vi "PID_TUNING.vi"() -> ()   [LabVIEW 2014]
doc: "This example performs writes and reads on a serial port, as directed by the user. You can press the Write and Read buttons, and change the Read Count, while the example is running.\n\nThe parameters set for the serial port must match the parameters of the connected instrument or device. In this example, the Read Count parameter specifies the number of bytes that the serial port reads. If there were more bytes at the port than the specified number, those bytes would not be read. If there were less bytes at the port than the specified number, you would receive a timeout error.\n\nThis example expands upon the flow control options for XON and XOFF, allowing the user to choose those control characters. Also, the user can enable or disable a termination character. Some devices require a termination character in order to identify the end of command strings. Some devices send a termination character to signify the end of data to be read. This example shows how you can end the Read operation once a termination character is detected in the buffer and/or append a termination character at the end of the Write data."
uses:
  PID Mode.ctl
  InputSimulationMode.ctl
  Serial - Settings.ctl
  Parameters.ctl
  <vilib>/Instr/_visa.llb/VISA Configure Serial Port (Instr).vi
panel:
  in  "Tab Control":enum32{"Main", "Debug"}(tab)
  out "PWM":u16(slide) scale=0.0..1023.0
  in  "Enable Commands":bool
  in  "Sync Commands":bool
  out "Input Mode Actual":T1
  in  "Input Mode":T1
  in  "COM Port":refnum<visa-resource-name>="COM1"
  in  "Stop":bool
  in  "Command Cluster":T2={"Setpoint"=0.0, "Temp C"=0.0, "Output"=0, "kP"=40.0, "kI"=1.0, "Kd"=0.1} {"Kd" scale=0.0..5.0; "kI" scale=0.0..10.0; "kP" scale=0.0..40.0; "Output" scale=0.0..961.0; "Temp C" scale=0.0..500.0; "Setpoint" scale=0.0..500.0}
  out "Setpoint":sgl(slide) scale=0.0..500.0
  out "Temp C":sgl(slide) scale=0.0..500.0
  out "Output":sgl(slide) scale=0.0..961.0
  out "kP":sgl(slide) scale=0.0..5.0
  out "kI":sgl(slide) scale=0.0..10.0
  out "Kd":sgl(slide) scale=0.0..5.0
  out "Waveform Chart":T3(graph)
  in  "PID Mode":T4
  out "PID Mode Actual":T4
  out "read buffer":string
  out "read buffer 2":string
  out "Start_of_packet":u8 format="%x"
  out "error out":errorcluster
  in  "Idle Temp C":i16
  out "Idle Temp C 2":i16
  out "Output Override":i16
  out "Simulated Tip Temp":sgl
  out "Command":string="*IDN?"
  out "adc_counts":i16
  out "Encoder Pos":i16
  out "adc_counts 2":i16
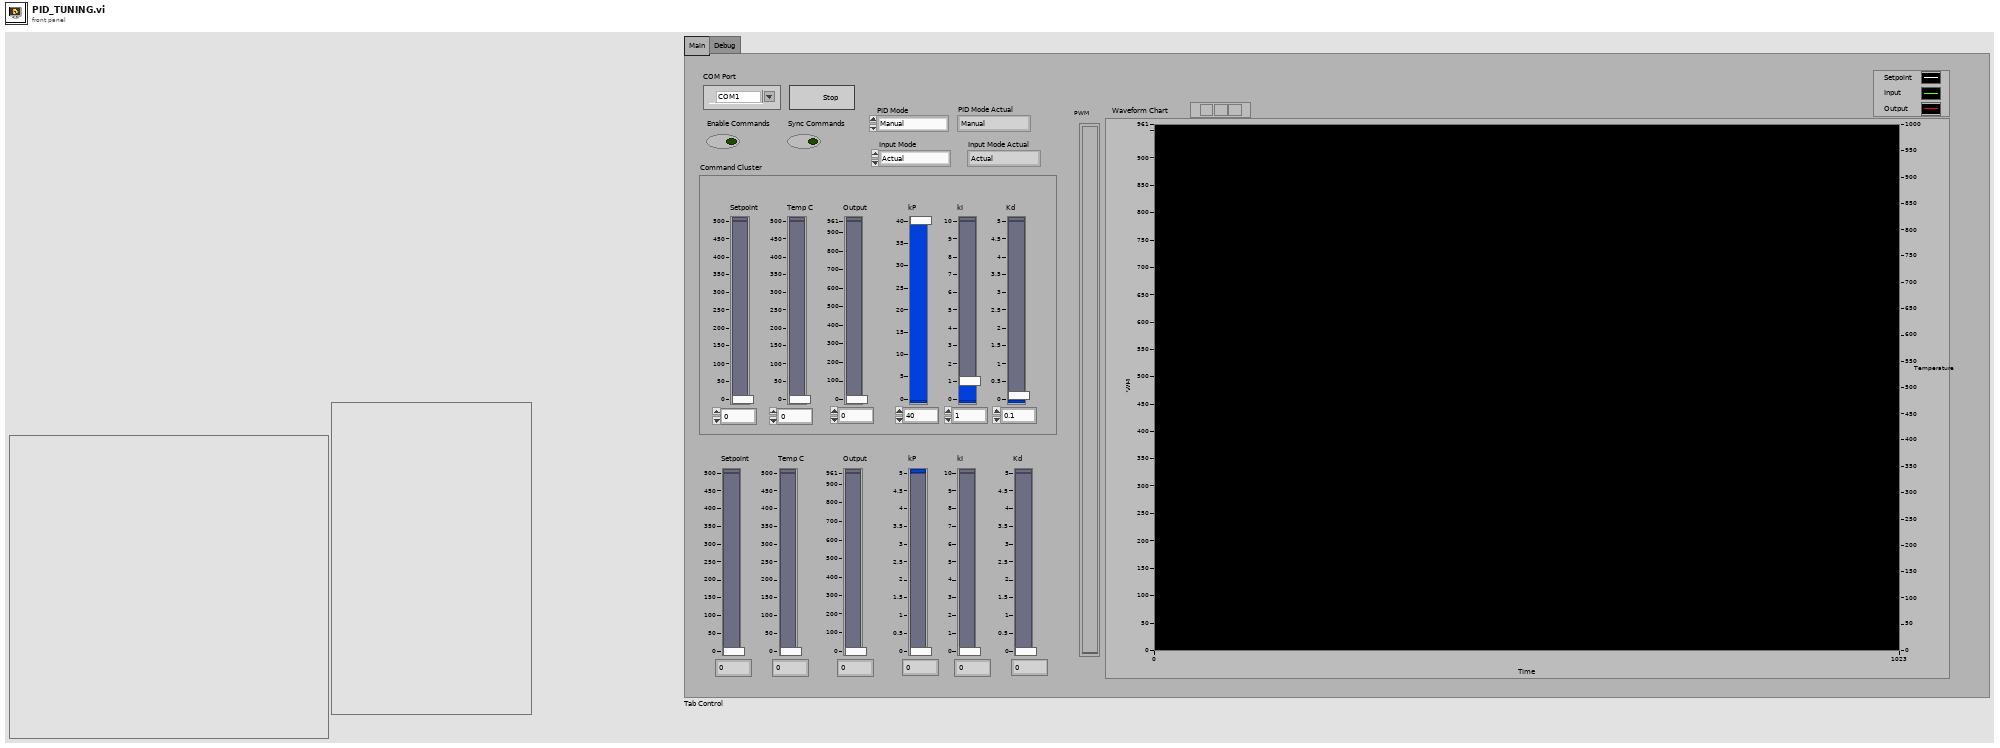
[diagram p1: front panel]
types:
  T1 = typedef "InputSimulationMode.ctl" = enum8{"Actual", "Simulated"}
  T2 = cluster{"Setpoint":sgl, "Temp C":sgl, "Output":i16, "kP":sgl, "kI":sgl, "Kd":sgl}
  T3 = cluster{"Setpoint":sgl, "Input":sgl, "Output":sgl}
  T4 = typedef "PID Mode.ctl" = enum8{"Manual", "Automatic"}
  T5 = typedef "Parameters.ctl" = cluster{"PID Mode":T4, "Input Mode":T1, "Idle Temp C":i16, "Output Override":i16, "setpoint":sgl, "kP":sgl, "kI":sgl, "kD":sgl, "Simulated Tip Temp C":sgl}
  T6 = typedef "Serial - Settings.ctl" = cluster{"baud rate":u32, "data bits":u16, "parity":enum16{"None", "Odd", "Even", "Mark", "Space"}, "stop bits":u16, "flow control":u16}
  T7 = typedef "Status.ctl" = cluster{"IO":bool[], "Encoder Pos":i16, "adapter voltage":i16, "adc_counts":i16, "adc_ic_temp_counts":i16, "current_sense_mv":i16, "PID Setpoint":sgl, "Tip Temp C":sgl, "PID Output":sgl}
  T8 = cluster{"PID Setpoint":sgl, "Tip Temp C":sgl, "PID Output":sgl}
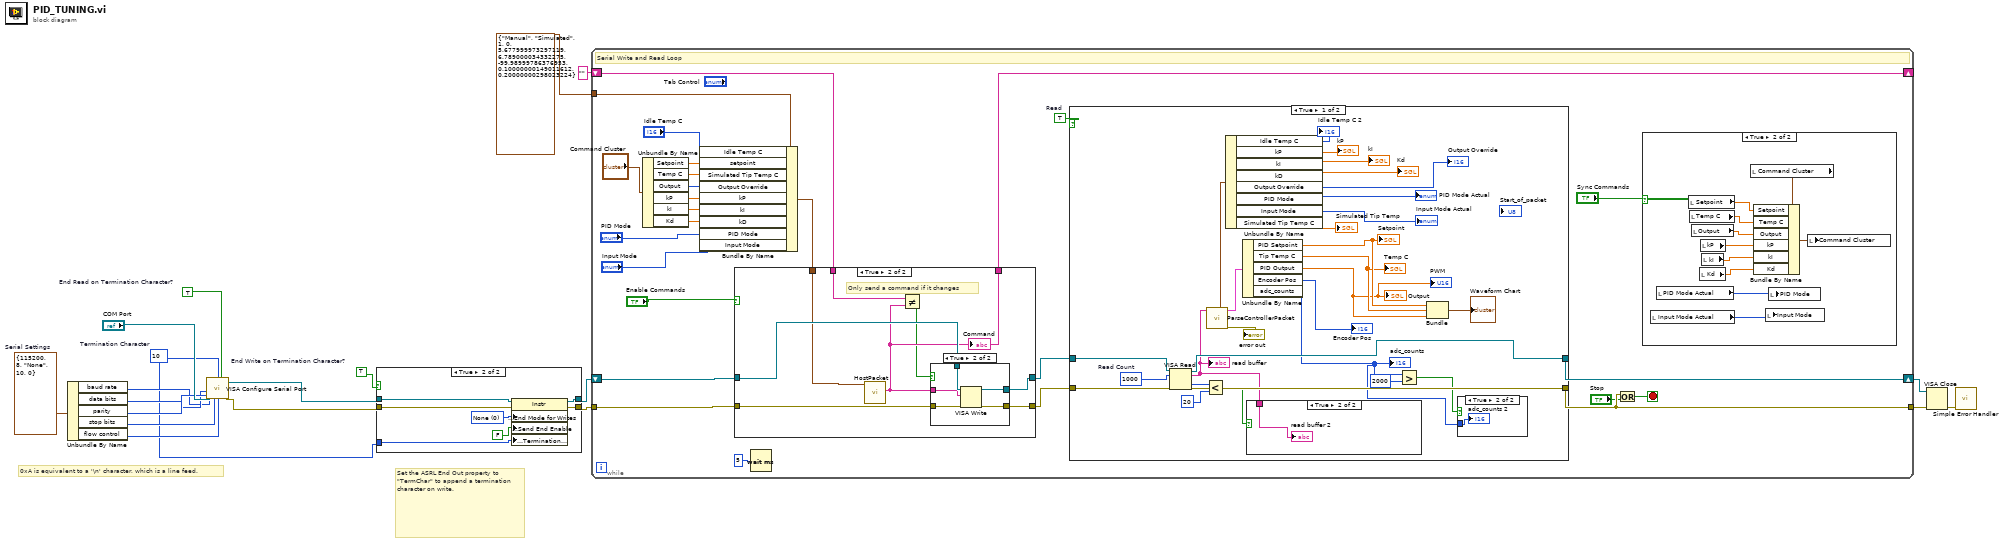
[diagram p0: block diagram]
diagram:
  w3 = u8 10  # Termination Character
  w4 = TRUE  # End Write on Termination Character?
  w11 = TRUE  # End Read on Termination Character?
  w12 = T6 {"baud rate"=115200, "data bits"=8, "parity"=enum."None", "stop bits"=10, "flow control"=0}  # Serial Settings
  # "0xA is equivalent to a '\\n' character, which is a line feed."
  # "Set the ASRL End Out property to \"TermChar\" to append a termination character on write."
  n1 = Unbundle By Name(w12) -> ("baud rate"=w13:u32, "data bits"=w14:u16, "parity"=w15:enum16{"None", "Odd", "Even", "Mark", "Space"}, "stop bits"=w16:u16, "flow control"=w7:u16)
  n2 = call-poly "VISA Configure Serial Port"("VISA resource name"="COM Port", "termination char\n(0xA = '\\n' = LF)"=w3, "Enable Termination\nChar (T)"=w11, "baud rate (9600)"=w13, "data bits (8)"=w14, "parity (0:none)"=w15, "stop bits (10: 1 bit)"=w16, "flow control (0:none)"=w7) -> ("VISA resource name out"=w17:refnum<visa-resource-name>, "error out"=w18:errorcluster)  [unwired: 2 in, 4 out]
  n3 = case shown="True" w4 {
    tunnel: w17 -> [w20 w28]
    tunnel: w18 -> [w21 w27]
    tunnel: [w20 w26] -> w5
    tunnel: [w21 w25] -> w6
    tunnel: w3 -> [_ w23]
    frame False {
    }
    frame True {
      w24 = u16 0 items=["None", "LastBit", "TermChar", "Break"] ("Serial Settings:Serial End Mode for Writes")
      n4 = property class="Instr"(reference=w28, error in=w27, "Serial Settings:End Mode for Writes"=w24, "Message Based Settings:Send End Enable"=FALSE, "Message Based Settings:Termination Character"=w23) -> (reference out=w26:refnum<visa-resource-name>, error out=w25:errorcluster)
    }
  }
  n5 = while {
    shift-right: [w54] -> w8
    shift-left: w5 -> [w53]
    tunnel: w6 -> [w52]
    tunnel: [w46] -> w9
    shift-right: [w44] -> _
    shift-left: "" ("string") -> [w43]
    tunnel: T5 {"PID Mode"=enum."Manual", "Input Mode"=enum."Simulated", "Idle Temp C"=1, "Output Override"=0, "setpoint"=5.678, "kP"=6.789, "kI"=-99.99, "kD"=0.1, "Simulated Tip Temp C"=0.2} ("Parameters") -> [w40]
    stop <- w47 stop-if-true
    w48 = TRUE  # Read
    # "Serial Write and Read Loop"
    n6 = Unbundle By Name("Command Cluster") -> ("Setpoint"=w41:sgl, "Temp C"=w39:sgl, "Output"=w38:i16, "kP"=w37:sgl, "kI"=w36:sgl, "Kd"=w35:sgl)
    n7 = Bundle By Name(cluster=w40, "Idle Temp C"="Idle Temp C", "setpoint"=w41, "Simulated Tip Temp C"=w39, "Output Override"=w38, "kP"=w37, "kI"=w36, "kD"=w35, "PID Mode"="PID Mode", "Input Mode"="Input Mode") -> (w32:T5)
    n8 = case shown="True" "Enable Commands" {
      tunnel: w53 -> [w67 w75]
      tunnel: w52 -> [w66 w74]
      tunnel: [w67 w73] -> w51
      tunnel: [w66 w72] -> w50
      tunnel: [w65 w70] -> w44
      tunnel: w43 -> [w65 w71]
      tunnel: w32 -> [_ w68]
      frame False {
      }
      frame True {
        # "Only send a command if it changes"
        n9 = call "HostPacket.vi"("Parameters"=w68) -> ("string"=w70:string)  [unwired: 9 in, 1 out]
        "Command" <- w70
        n10 = Not Equal?(x=w71, y=w70) -> (x != y?=w69:bool)
        n11 = case shown="True" w69 {
          tunnel: w75 -> [w76 w82]
          tunnel: w74 -> [w77 w81]
          tunnel: [w76 w80] -> w73
          tunnel: [w77 w79] -> w72
          tunnel: w70 -> [_ w78]
          frame False {
          }
          frame True {
            n12 = VISA Write(VISA resource name=w82, write buffer=w78, error in (no error)=w81) -> (VISA resource name out=w80:refnum<visa-resource-name>, error out=w79:errorcluster)  [unwired: 1 out]
          }
        }
      }
    }
    n13 = Wait (ms)(milliseconds to wait=u32 5) -> ()  [unwired: 1 out]
    n14 = case shown="True" w48 {
      tunnel: [w108 w114] -> w54
      tunnel: w51 -> [w110 w114]
      tunnel: [w106 w113] -> w46
      tunnel: w50 -> [w109 w113]
      frame True {
        w107 = u32 1000  # Read Count
        n15 = VISA Read(VISA resource name=w110, byte count=w107, error in (no error)=w109) -> (VISA resource name out=w108:refnum<visa-resource-name>, read buffer=w101:string, return count=w105:u32, error out=w106:errorcluster)
        "read buffer" <- w101
        n16 = Less?(x=w105, y=u32 20) -> (x < y?=w103:bool)
        n17 = call "ParseControllerPacket.vi"("Hex String"=w101) -> ("error out"=→"error out":errorcluster, "Status"=w100:T7, "Parameters"=w96:T5)  [unwired: 8 in]
        n18 = Unbundle By Name(w96) -> ("Idle Temp C"=→"Idle Temp C 2":i16, "kP"=→"kP":sgl, "kI"=→"kI":sgl, "kD"=→"Kd":sgl, "Output Override"=→"Output Override":i16, "PID Mode"=→"PID Mode Actual":T4, "Input Mode"=→"Input Mode Actual":T1, "Simulated Tip Temp C"=→"Simulated Tip Temp":sgl)
        n19 = Unbundle By Name(w100) -> ("PID Setpoint"=w99:sgl, "Tip Temp C"=w97:sgl, "PID Output"=w83:sgl, "Encoder Pos"=→"Encoder Pos":i16, "adc_counts"=w84:i16)
        "Setpoint" <- w99
        "Temp C" <- w97
        "Output" <- w83
        "adc_counts" <- w84
        "PWM" <- w83
        n20 = case shown="True" w103 {
          tunnel: w101 -> [_ w112]
          frame False {
          }
          frame True {
            "read buffer 2" <- w112
          }
        }
        n21 = Greater?(x=w84, y=i16 2000) -> (0:w85:bool)
        n22 = Bundle("PID Setpoint"=w99, "Tip Temp C"=w97, "PID Output"=w83) -> (→"Waveform Chart":T8)  [unwired: 1 in]
        n23 = case shown="True" w85 {
          tunnel: w84 -> [_ w111]
          frame False {
          }
          frame True {
            "adc_counts 2" <- w111
          }
        }
      }
      frame False {
      }
    }
    n24 = Or(x=w46, y="Stop") -> (x .or. y?=w47:bool)
    n25 = case shown="True" "Sync Commands" {
      frame False {
      }
      frame True {
        n26 = local read "Input Mode Actual"() -> (w55:T1)
        n27 = local read "PID Mode Actual"() -> (w56:T4)
        n28 = local read "Setpoint"() -> (w62:sgl)
        n29 = local read "Temp C"() -> (w61:sgl)
        n30 = local read "Output"() -> (w60:sgl)
        n31 = local read "Kd"() -> (w57:sgl)
        n32 = local read "kP"() -> (w59:sgl)
        n33 = local read "kI"() -> (w58:sgl)
        n34 = local read "Command Cluster"() -> (w64:T2)
        n35 = Bundle By Name(cluster=w64, "Setpoint"=w62, "Temp C"=w61, "Output"=w60, "kP"=w59, "kI"=w58, "Kd"=w57) -> (w63:T2)
        n36 = local write "Input Mode"(w55) -> ()
        n37 = local write "PID Mode"(w56) -> ()
        n38 = local write "Command Cluster"(w63) -> ()
      }
    }
  }
  n39 = VISA Close(VISA resource name=w8, error in (no error)=w9) -> (error out=w10:errorcluster)
  n40 = call <vilib>:"Simple Error Handler.vi"("error in (no error)"=w10) -> ()  [unwired: 1 in, 8 out]
